vi "Pockels Cal-Cleanup.vi"(6 "Pockels calibration voltage steps sequence (strings)":string[](array[string])=["0.0", "0.1", "0.2", "0.3", "0.4", "0.5", "0.6", "0.7", "0.8", "0.9", "1.0", "1.1", "1.2", "1.3", "1.4", "1.5", "1.6", "1.7", "1.8", "1.9", "2.0"], 8 "error in (no error)":errorcluster, 9 "Timed out or error":bool, 10 "Cancelled/Aborted":bool, 11 "Calibration data (all objectives even if blank)":string[][](array[string])=[["No objective", "0", "1.0", "1.0", "1.0", "1.0", "1.0", "1.0", "1.0", "1.0", "1.0", "1.0", "1.0", "1.0", "1.0", "1.0", "1.0", "1.0", "1.0", "1.0", "1.0", "1.0"], ["Olympus 20X", "", "", "", "", "", "", "", "", "", "", "", "", "", "", "", "", "", "", "", "", ""], ["Nikon 25X", "", "", "", "", "", "", "", "", "", "", "", "", "", "", "", "", "", "", "", "", ""], ["Olympus 40X", "", "", "", "", "", "", "", "", "", "", "", "", "", "", "", "", "", "", "", "", ""], ["Olympus 60X", "", "", "", "", "", "", "", "", "", "", "", "", "", "", "", "", "", "", "", "", ""]]) -> (0 "error out":errorcluster, 1 "Timed out or errored out":bool, 2 "Formatted cal table (inc. header)":string[][](array[string]), 3 "VI out":refnum<vi>, 4 "Cancelled/Aborted":bool)   [LabVIEW 2013]
uses:
  Peripherals Control/Shutter/Typedefs/Shutter state.ctl
  Typedefs/Functional global standard states.ctl
  Globals/gl_Calibration globals.vi
  Global Variables/gl_UI Ctrl Refs.vi
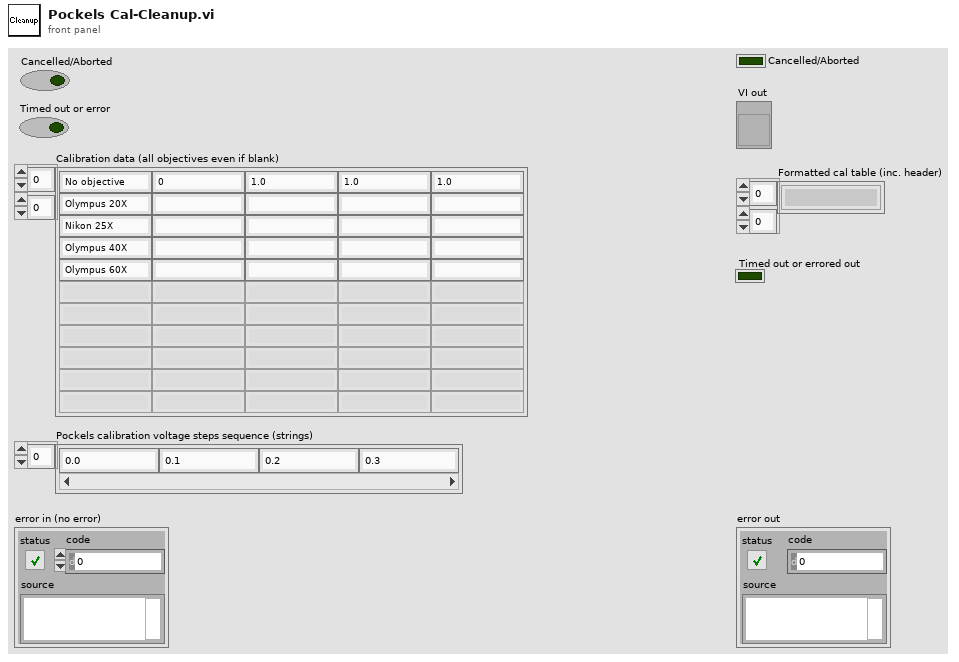
[diagram p1: front panel]
types:
  T1 = enum32{"Invalid", "Standard", "Closed", "Hidden", "Minimized", "Maximized"}
  T2 = typedef "Pockels cal process refs.ctl" = cluster{"This VI":refnum<vi>, "Abort (ind)":refnum<vi>, "Next (ind)":refnum<vi>, "Cancel":refnum<vi>, "Next":refnum<vi>, "Message":refnum<vi>, "Measured Power ctrl":refnum<vi>, "Measured Power ind":refnum<vi>, "Pockels cal progress bar":refnum<vi>, "Abort this objective":refnum<vi>}
  T3 = typedef "Shutter state.ctl" = enum16{"Closed/Disabled", "Open/Enabled"}
  T4 = typedef "Functional global standard states.ctl" = enum16{"Initialise", "Read", "Write", "Load", "Save", "Clear"}
  T5 = typedef "UI ctrl refs cluster.ctl" = cluster{"Top level VI path":path, "Top level VI ref":refnum<vi>, "User menu ref":refnum<k9>, "Sub Panel control":refnum<vi>, "Imaging Param Tab":refnum<vi>, "Occurrence-Start drivers":refnum<k4>, "Occurrence-Speed logging initialised":refnum<k4>, "Occurrence-XYZ stage initialised":refnum<k4>, "Exit button":refnum<vi>, "Status ind":refnum<vi>, "Return to Origin":refnum<vi>, "Speed Logging":refnum<vi>, "Time Lapse":refnum<vi>, "Live Imaging":refnum<vi>, "AOL Z Stack":refnum<vi>, "Motor Z Stack":refnum<vi>, "Funct Acq button":refnum<vi>, "Hard Shutter":refnum<vi>, "Virtual Shutter":refnum<vi>, "Laser Power":refnum<vi>, "AOL Mode":refnum<vi>, "Frame Size":refnum<vi>, "Field of View":refnum<vi>, "Dwell Time":refnum<vi>, "Zoom":refnum<vi>, "AOL Z":refnum<vi>, "Objective":refnum<vi>, "Axis":refnum<vi>, "Paths & Names":refnum<vi>, "Experiment folder path (ind.)":refnum<vi>, "Last State (Ind.)":refnum<vi>, "Laser wavelength ind (nm)":refnum<vi>, "Averages":refnum<vi>, "Angle (degrees)":refnum<vi>, "X centre":refnum<vi>, "Y centre":refnum<vi>, "Plane Mode":refnum<vi>, "# Planes":refnum<vi>, "Z Start":refnum<vi>, "Z Stop":refnum<vi>, "Z Step":refnum<vi>, "PMT 1":refnum<vi>, "PMT 2":refnum<vi>, "Stage XYZ Position":refnum<vi>, "Pockels@Z Start":refnum<vi>, "Pockels@Z Stop":refnum<vi>, "Obtain Z Start":refnum<vi>, "Obtain Z Stop":refnum<vi>, "Live stim.trig.period":refnum<vi>, "Live stim.trig.enable":refnum<vi>, "Funct. Acq. Pockels Modulation":refnum<vi>, "Enable Video Recording":refnum<vi>, "Video Record-Live Imaging":refnum<vi>, "Video Record-Funct acq":refnum<vi>, "AOL Z-stack Chirps Ready (ind)":refnum<vi>, "Center freq ind (nm)":refnum<vi>, "Logging queue (ind)":refnum<vi>, "Back aperture power (ind.)":refnum<vi>, "Power after objective (ind.)":refnum<vi>, "Switch user":refnum<vi>}
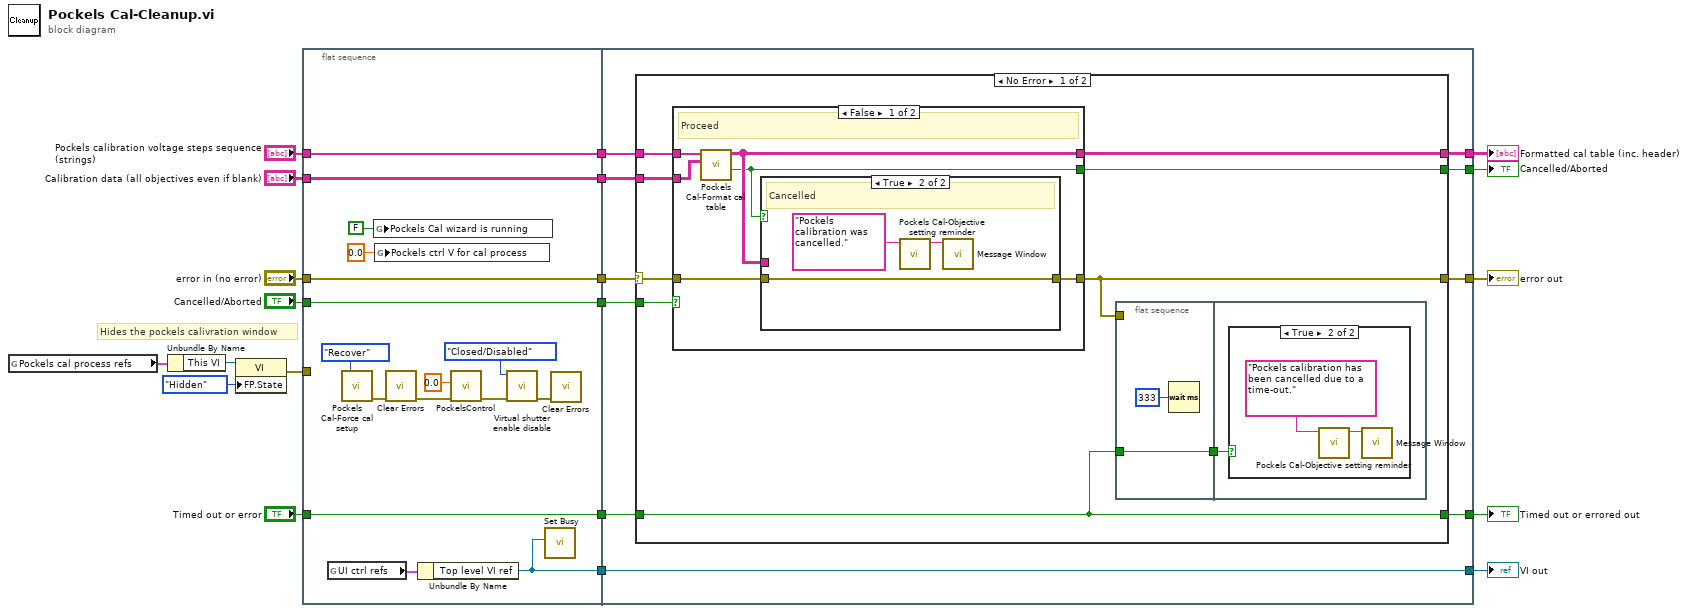
[diagram p0: block diagram]
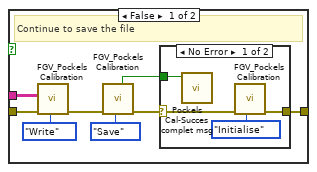
[diagram p3: hidden frame]
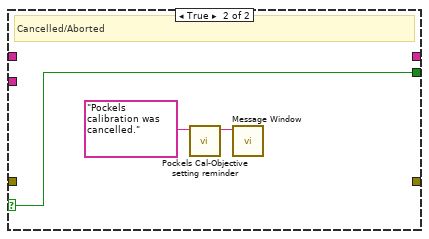
[diagram p5: hidden frame]
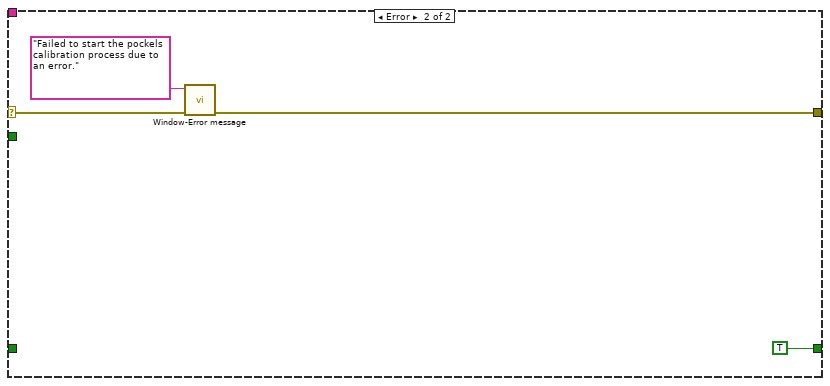
[diagram p6: hidden frame]
diagram:
  # "Hides the pockels calivration window"
  n1 = global read "gl_Calibration globals.vi" "Pockels cal process refs"() -> (w5:T2)
  n2 = Unbundle By Name(w5) -> ("This VI"=w4:refnum<vi>)
  n3 = property class="VI"(reference=w4, "FP.State"=T1."Hidden" ("Front Panel Window:State")) -> (error out=w2:errorcluster)  [unwired: 1 in, 1 out]
  n4 = flat-sequence {
    tunnel: "Pockels calibration voltage steps sequence (strings)" -> [w32]
    tunnel: "error in (no error)" -> [w33]
    tunnel: "Cancelled/Aborted" -> [w34]
    tunnel: "Timed out or error" -> [w35]
    tunnel: "Calibration data (all objectives even if blank)" -> [w36]
    tunnel: [w36] -> w20
    tunnel: [w35] -> w19
    tunnel: [w34] -> w18
    tunnel: [w33] -> w17
    tunnel: [w32] -> w16
    tunnel: [w26] -> w15
    tunnel: w2 -> [_]
    tunnel: [w40] -> w9
    tunnel: w20 -> [w46]
    tunnel: w19 -> [w43]
    tunnel: w18 -> [w41]
    tunnel: w17 -> [w39]
    tunnel: w16 -> [w45]
    tunnel: w15 -> [w42]
    tunnel: [w44] -> w12
    tunnel: [w37] -> w13
    tunnel: [w42] -> w14
    tunnel: [w38] -> w1
    frame #0 {
      n5 = global read "gl_UI Ctrl Refs.vi" "UI ctrl refs"() -> (w28:T5)
      n6 = call "Pockels Cal-Force cal setup.vi"("Function"=enum16{"Set", "Recover"}."Recover") -> ("error out"=w27:errorcluster)  [unwired: 10 in]
      n7 = global write "gl_Calibration globals.vi" "Pockels Cal wizard is running"(FALSE ("Motor Z Cal wizard is running")) -> ()
      n8 = global write "gl_Calibration globals.vi" "Pockels ctrl V for cal process"(0.0 ("Norm coord for cal process")) -> ()
      n9 = call <vilib>:"Clear Errors.vi"("error in (no error)"=w27) -> ("error out"=w22:errorcluster)  [unwired: 6 in]
      n10 = Unbundle By Name(w28) -> ("Top level VI ref"=w26:refnum<vi>)
      n11 = call "PockelsControl.vi"("Error In"=w22, "Laser Power (%)"=0.0) -> ("Error Out"=w24:errorcluster)  [unwired: 9 in]
      n12 = call "Virtual shutter enable disable.vi"("error in (no error)"=w24, "Virtual Shutter"=Shutter_state."Closed/Disabled") -> ("error out"=w21:errorcluster)  [unwired: 9 in]
      n13 = call <vilib>:"Set Busy.vi"("VI reference (current VI)"=w26) -> ()  [unwired: 9 in, 2 out]
      n14 = call <vilib>:"Clear Errors.vi"("error in (no error)"=w21) -> ()  [unwired: 6 in, 1 out]
    }
    frame #1 {
      n15 = case shown="No Error" w39 {
        selector: w39 -> [w50 w88]
        tunnel: w46 -> [w54 _]
        tunnel: w45 -> [w53 _]
        tunnel: [w52 _] -> w44
        tunnel: w43 -> [w48 _]
        tunnel: w41 -> [w51 _]
        tunnel: [w47 w87] -> w40
        tunnel: [w49 _] -> w38
        tunnel: [w48 TRUE] -> w37
        frame No Error {
          n16 = case shown="False" w51 {
            selector: w51 -> [_ w85]
            tunnel: w53 -> [w63 _]
            tunnel: w54 -> [w66 _]
            tunnel: [w65 _] -> w47
            tunnel: [w64 _] -> w52
            tunnel: w50 -> [w62 _]
            tunnel: [w61 w85] -> w49
            frame False {
              # "Proceed"
              n17 = call "Pockels Cal-Format cal table.vi"("Calibration data (all objectives even if blank + inc. data header row)"=w66, "Pockels calibration voltage steps sequence (1st column)"=w63) -> ("Cancelled"=w61:bool, "Formatted cal table (inc. header)"=w64:string[][])  [unwired: 8 in]
              n18 = case shown="True" w61 {
                tunnel: [w68 w82] -> w65
                tunnel: w64 -> [w74 _]
                tunnel: w62 -> [w70 w82]
                frame False {
                  # "Continue to save the file"
                  n19 = call "FGV_Pockels Calibration.vi"("error in (no error)"=w70, "Function"=Functional_global_standard_states."Write", "Pockels Cal table (Single wavelength)"=w74) -> ("error out"=w72:errorcluster)  [unwired: 2 in, 6 out]
                  n20 = call "FGV_Pockels Calibration.vi"("error in (no error)"=w72, "Function"=Functional_global_standard_states."Save") -> ("error out"=w69:errorcluster, "Updated existing file?"=w67:bool)  [unwired: 3 in, 5 out]
                  n21 = case shown="No Error" w69 {
                    selector: w69 -> [w76 w79]
                    tunnel: [w75 w79] -> w68
                    tunnel: w67 -> [w78 _]
                    frame No Error {
                      n22 = call "Pockels Cal-Succes complet msg.vi"("Updated existing file?"=w78) -> ()  [unwired: 10 in, 1 out]
                      n23 = call "FGV_Pockels Calibration.vi"("error in (no error)"=w76, "Function"=Functional_global_standard_states."Initialise") -> ("error out"=w75:errorcluster)  [unwired: 3 in, 6 out]
                    }
                    frame Error {
                    }
                  }
                }
                frame True {
                  # "Cancelled"
                  n24 = call "Pockels Cal-Objective setting reminder.vi"("Message in"="Pockels calibration was cancelled." ("Message string")) -> ("Message"=w80:string)  [unwired: 10 in]
                  n25 = call "Message Window.vi"("Message string"=w80) -> ()  [unwired: 10 in, 1 out]
                }
              }
            }
            frame True {
              # "Cancelled/Aborted"
              n26 = call "Pockels Cal-Objective setting reminder.vi"("Message in"="Pockels calibration was cancelled." ("Message string")) -> ("Message"=w84:string)  [unwired: 10 in]
              n27 = call "Message Window.vi"("Message string"=w84) -> ()  [unwired: 10 in, 1 out]
            }
          }
          n28 = flat-sequence {
            tunnel: w48 -> [w57]
            tunnel: [w57] -> w55
            tunnel: w47 -> [_]
            tunnel: w55 -> [w58]
            frame #0 {
              n29 = Wait (ms)(milliseconds to wait=u32 333) -> ()  [unwired: 1 out]
            }
            frame #1 {
              n30 = case shown="True" w58 {
                frame False {
                }
                frame True {
                  n31 = call "Pockels Cal-Objective setting reminder.vi"("Message in"="Pockels calibration has been cancelled due to a time-out." ("Message string")) -> ("Message"=w59:string)  [unwired: 10 in]
                  n32 = call "Message Window.vi"("Message string"=w59) -> ()  [unwired: 10 in, 1 out]
                }
              }
            }
          }
        }
        frame Error {
          n33 = call "Window-Error message.vi"("error in (no error)"=w88, "Message"="Failed to start the pockels calibration process due to an error." ("Error Message")) -> ("Error Out (no error)"=w87:errorcluster)  [unwired: 9 in]
        }
      }
    }
  }
  "VI out" <- w14
  "Timed out or errored out" <- w13
  "Formatted cal table (inc. header)" <- w12
  "error out" <- w9
  "Cancelled/Aborted" <- w1
